vi "Debounce.vi"(6 "Time Threshold":u32, 8 "Default Value":bool, 11 "Boolean In":bool) -> (3 "Boolean Out":bool)   [LabVIEW 2012]
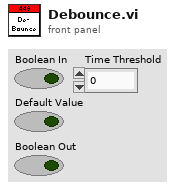
[diagram p1: front panel]
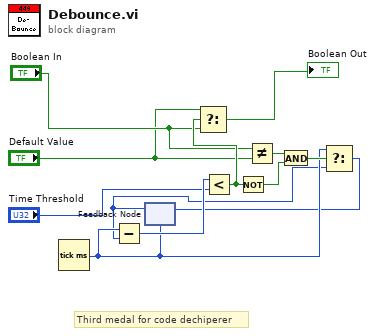
[diagram p0: block diagram]
diagram:
  # "Third medal for code dechiperer"
  n1 = Tick Count (ms)() -> (millisecond timer value=w3:u32)
  n2 = feedback #1(w3) -> (w2:u32)
  n3 = Subtract(x=w3, y=w2) -> (x-y=w12:u32)
  n4 = Less?(x=w12, y="Time Threshold") -> (x < y?=w9:bool)
  n5 = Select(t="Default Value", s=w9, f="Boolean In") -> (s? t:f=→"Boolean Out":bool)
  n6 = Not(x=w9) -> (.not. x?=w5:bool)
  n7 = Not Equal?(x="Boolean In", y="Default Value") -> (x != y?=w6:bool)
  n8 = And(x=w6, y=w5) -> (x .and. y?=w4:bool)
  n9 = Select(t=w3, s=w4, f=w2) -> (s? t:f=w1:u32)
  n10 = feedback-in #1(w1) -> ()
